vi "start accessory panels.vi"(8 "error in (no error)":errorcluster, 9 "stim laser ref":refnum<vi>, 10 "FPGA VI ref":T1, 11 "Queues":T3) -> (0 "error out":errorcluster, 3 "refs":T2)   [LabVIEW 2010]
uses:
  internal_queues.ctl
  line_info.ctl
  volume_with_lines.ctl
  volume_info.ctl
  kalman_result_scaled.ctl
  location3D.ctl
  FPGA_ref.ctl
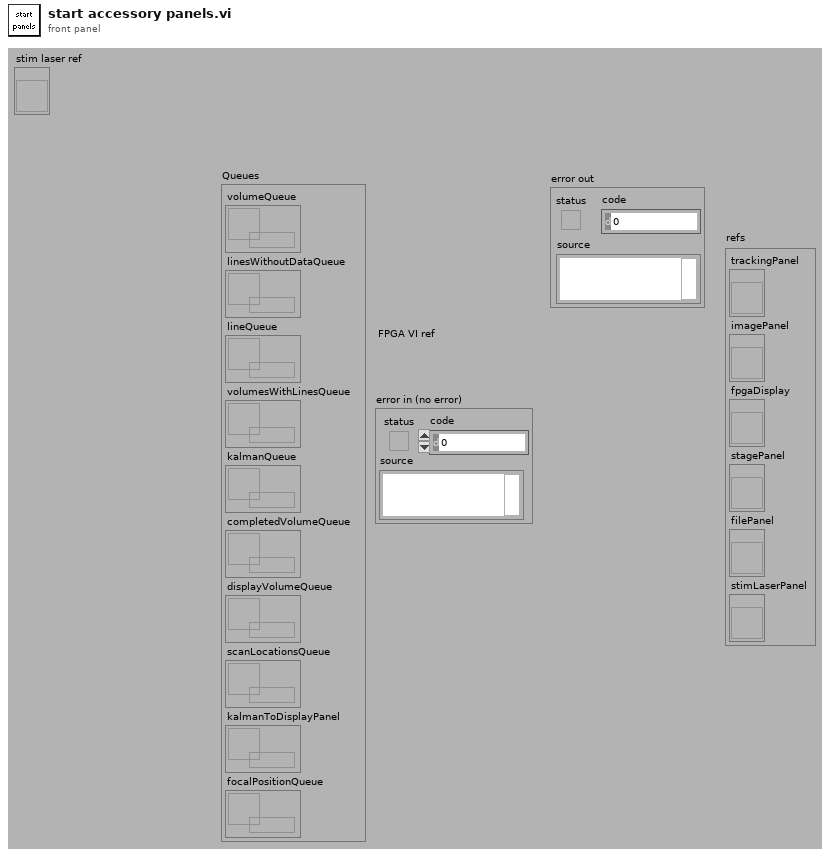
[diagram p1: front panel]
types:
  T1 = typedef "FPGA_ref.ctl" = refnum<k20>
  T2 = cluster{"trackingPanel":refnum<vi>, "imagePanel":refnum<vi>, "fpgaDisplay":refnum<vi>, "stagePanel":refnum<vi>, "filePanel":refnum<vi>, "stimLaserPanel":refnum<vi>}
  T3 = typedef "internal_queues.ctl" = cluster{"volumeQueue":refnum<queue>, "linesWithoutDataQueue":refnum<queue>, "lineQueue":refnum<queue>, "volumesWithLinesQueue":refnum<queue>, "kalmanQueue":refnum<queue>, "completedVolumeQueue":refnum<queue>, "displayVolumeQueue":refnum<queue>, "scanLocationsQueue":refnum<queue>, "kalmanToDisplayPanel":refnum<queue>, "focalPositionQueue":refnum<queue>}
  T4 = cluster{refnum<vi>, refnum<vi>, refnum<vi>, refnum<vi>, refnum<vi>, refnum<vi>}
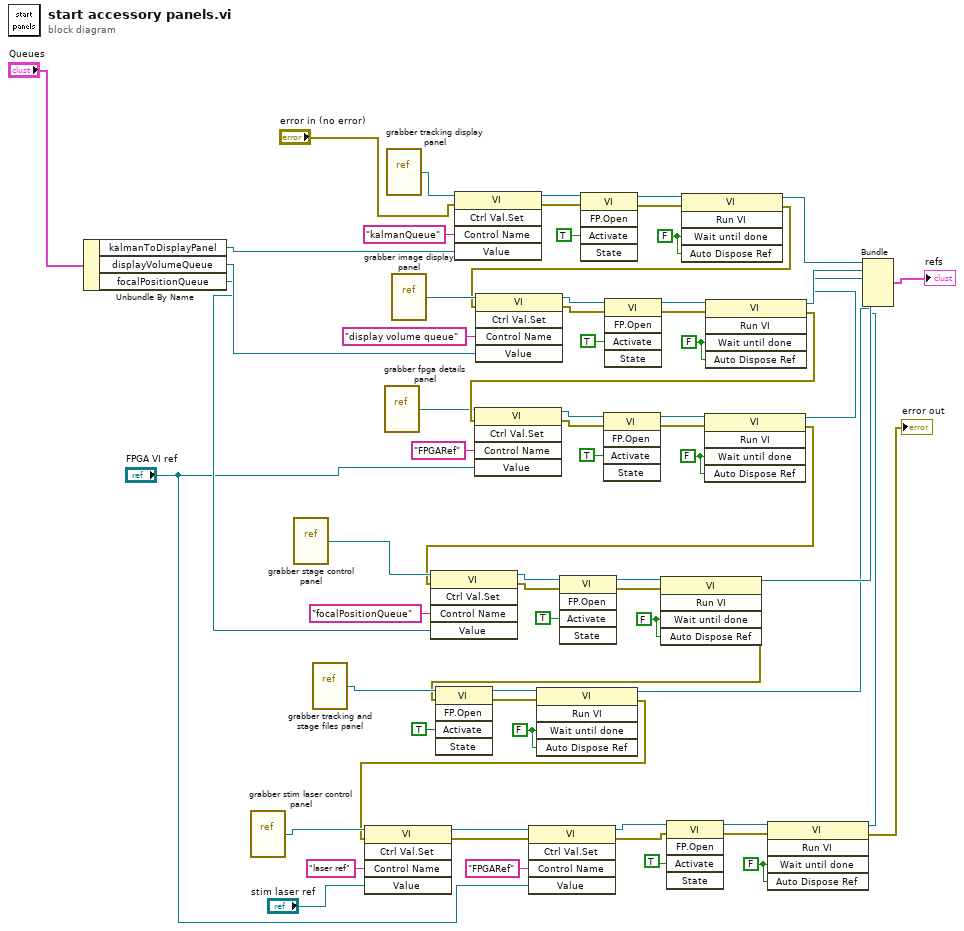
[diagram p0: block diagram]
diagram:
  w15 = FALSE ("Wait Until Done")
  w20 = FALSE ("Wait Until Done")
  w28 = FALSE ("Wait Until Done")
  w38 = FALSE ("Wait Until Done")
  w55 = FALSE ("Wait Until Done")
  w62 = FALSE ("Wait Until Done")
  n1 = Unbundle By Name("Queues") -> ("kalmanToDisplayPanel"=w66:refnum<queue>, "displayVolumeQueue"=w52:refnum<queue>, "focalPositionQueue"=w25:refnum<queue>)
  n2 = vi-ref "grabber stim laser control panel.vi"() -> (w12:refnum<vi>)
  n3 = vi-ref "grabber stage control panel.vi"() -> (w27:refnum<vi>)
  n4 = vi-ref "grabber tracking and stage files panel.vi"() -> (w19:refnum<vi>)
  n5 = vi-ref "grabber fpga details panel.vi"() -> (w35:refnum<vi>)
  n6 = vi-ref "grabber tracking display panel.vi"() -> (w51:refnum<vi>)
  n7 = vi-ref "grabber image display panel.vi"() -> (w49:refnum<vi>)
  n8 = invoke class="VI" method="Ctrl Val.Set"(reference=w51, error in="error in (no error)", "Control Name"="kalmanQueue", "Value"=w66) -> (reference out=w54:refnum<vi>, error out=w53:errorcluster)  [unwired: 1 in, 3 out]
  n9 = invoke class="VI" method="FP.Open"(reference=w54, error in=w53, "Activate"=TRUE ("Activate?")) -> (reference out=w63:refnum<vi>, error out=w64:errorcluster)  [unwired: 2 in, 3 out]
  n10 = invoke class="VI" method="Run VI"(reference=w63, error in=w64, "Wait until done"=w62, "Auto Dispose Ref"=w62) -> (reference out=w47:refnum<vi>, error out=w48:errorcluster)  [unwired: 1 in, 3 out]
  n11 = invoke class="VI" method="Ctrl Val.Set"(reference=w49, error in=w48, "Control Name"="display volume queue", "Value"=w52) -> (reference out=w60:refnum<vi>, error out=w59:errorcluster)  [unwired: 1 in, 3 out]
  n12 = invoke class="VI" method="FP.Open"(reference=w60, error in=w59, "Activate"=TRUE ("Activate?")) -> (reference out=w56:refnum<vi>, error out=w57:errorcluster)  [unwired: 2 in, 3 out]
  n13 = invoke class="VI" method="Run VI"(reference=w56, error in=w57, "Wait until done"=w55, "Auto Dispose Ref"=w55) -> (reference out=w46:refnum<vi>, error out=w37:errorcluster)  [unwired: 1 in, 3 out]
  n14 = invoke class="VI" method="Ctrl Val.Set"(reference=w35, error in=w37, "Control Name"="FPGARef", "Value"="FPGA VI ref") -> (reference out=w43:refnum<vi>, error out=w42:errorcluster)  [unwired: 1 in, 3 out]
  n15 = invoke class="VI" method="FP.Open"(reference=w43, error in=w42, "Activate"=TRUE ("Activate?")) -> (reference out=w39:refnum<vi>, error out=w40:errorcluster)  [unwired: 2 in, 3 out]
  n16 = invoke class="VI" method="Run VI"(reference=w39, error in=w40, "Wait until done"=w38, "Auto Dispose Ref"=w38) -> (reference out=w36:refnum<vi>, error out=w26:errorcluster)  [unwired: 1 in, 3 out]
  n17 = invoke class="VI" method="Ctrl Val.Set"(reference=w27, error in=w26, "Control Name"="focalPositionQueue", "Value"=w25) -> (reference out=w33:refnum<vi>, error out=w32:errorcluster)  [unwired: 1 in, 3 out]
  n18 = invoke class="VI" method="FP.Open"(reference=w33, error in=w32, "Activate"=TRUE ("Activate?")) -> (reference out=w29:refnum<vi>, error out=w30:errorcluster)  [unwired: 2 in, 3 out]
  n19 = invoke class="VI" method="Run VI"(reference=w29, error in=w30, "Wait until done"=w28, "Auto Dispose Ref"=w28) -> (reference out=w24:refnum<vi>, error out=w18:errorcluster)  [unwired: 1 in, 3 out]
  n20 = invoke class="VI" method="FP.Open"(reference=w19, error in=w18, "Activate"=TRUE ("Activate?")) -> (reference out=w21:refnum<vi>, error out=w22:errorcluster)  [unwired: 2 in, 3 out]
  n21 = invoke class="VI" method="Run VI"(reference=w21, error in=w22, "Wait until done"=w20, "Auto Dispose Ref"=w20) -> (reference out=w17:refnum<vi>, error out=w9:errorcluster)  [unwired: 1 in, 3 out]
  n22 = invoke class="VI" method="Ctrl Val.Set"(reference=w12, error in=w9, "Control Name"="laser ref", "Value"="stim laser ref") -> (reference out=w5:refnum<vi>, error out=w2:errorcluster)  [unwired: 1 in, 3 out]
  n23 = invoke class="VI" method="Ctrl Val.Set"(reference=w5, error in=w2, "Control Name"="FPGARef", "Value"="FPGA VI ref") -> (reference out=w4:refnum<vi>, error out=w3:errorcluster)  [unwired: 1 in, 3 out]
  n24 = invoke class="VI" method="FP.Open"(reference=w4, error in=w3, "Activate"=TRUE ("Activate?")) -> (reference out=w13:refnum<vi>, error out=w14:errorcluster)  [unwired: 2 in, 3 out]
  n25 = invoke class="VI" method="Run VI"(reference=w13, error in=w14, "Wait until done"=w15, "Auto Dispose Ref"=w15) -> (reference out=w7:refnum<vi>, error out=→"error out":errorcluster)  [unwired: 1 in, 3 out]
  n26 = Bundle(w47, w46, w36, w24, w17, w7) -> (→"refs":T4)  [unwired: 1 in]
